vi "PipelineDuty.vi"(8 "error in (no error)":errorcluster, 10 "DataExchange":T1, 11 "GRMActor in":refnum<class "DisplayerUI.lvclass">) -> (0 "error out":errorcluster, 2 "DataExchange Out":T1, 3 "GRMActor out":refnum<class "DisplayerUI.lvclass">)   [LabVIEW 2020, in "DisplayerUI.lvlib" / "DisplayerUI.lvclass"]
uses:
  DisplayerUI.lvclass
  Hardware Abstraction Layer/Component/Device/Device/DataExchange.ctl
  Hardware Abstraction Layer/Component/GenericActor/GenericActor/GenericController.lvclass
  DisplayerUI.lvclass/DisplayerUI.ctl
  Interface/DataListener/DataListener.lvclass
panel:
  out "Source":string
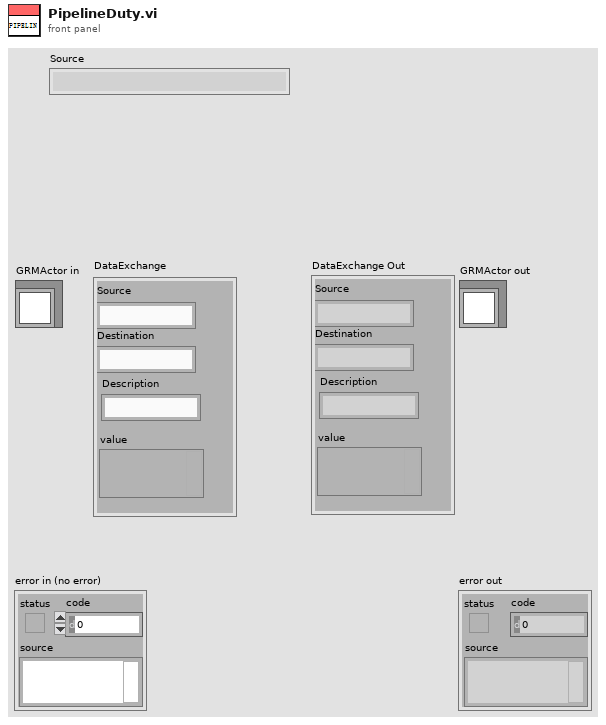
[diagram p1: front panel]
types:
  T1 = typedef "DataListener.lvclass/DataExchange.ctl" = cluster{"Source":string, "Destination":string, "Description":string, "value":variant}
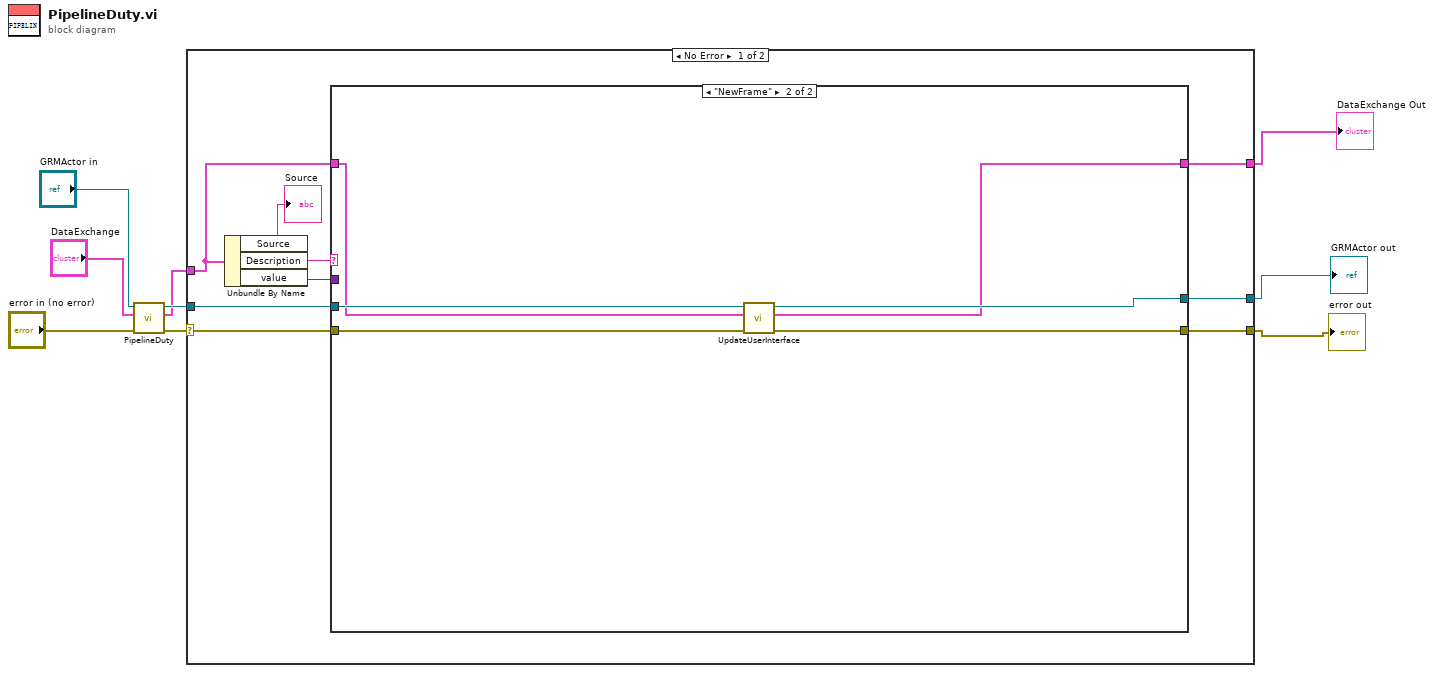
[diagram p0: block diagram]
diagram:
  n1 = call-parent "PipelineDuty.vi"("error in (no error)"="error in (no error)", "DataExchange"="DataExchange", "GRMActor in"="GRMActor in") -> ("error out"=w6:errorcluster, "DataExchange Out"=w4:T1, "GRMActor out"=w5:refnum<class "DisplayerUI.lvclass">)  [unwired: 6 in]
  n2 = case shown="No Error" w6 {
    selector: w6 -> [w16 w30]
    tunnel: [w17 w30] -> w2
    tunnel: w5 -> [w13 w29]
    tunnel: [w18 w29] -> w3
    tunnel: w4 -> [w12 w28]
    tunnel: [w11 w28] -> w1
    frame No Error {
      n3 = Unbundle By Name(w12) -> ("Source"=→"Source":string, "Description"=w15:string, "value"=w14:variant)
      n4 = case shown="\"NewFrame\"" w15 {
        tunnel: w14 -> [_ _]
        tunnel: [w21 w24] -> w18
        tunnel: w13 -> [w21 w25]
        tunnel: [w20 w26] -> w17
        tunnel: w16 -> [w20 w27]
        tunnel: w12 -> [w19 w23]
        tunnel: [w19 w22] -> w11
        frame Default {
        }
        frame "NewFrame" {
          n5 = call-dynamic "UpdateUserInterface.vi"("error in (no error)"=w27, "DataExchange"=w23, "DisplayerUI in"=w25) -> ("error out"=w26:errorcluster, "DataExchange Out"=w22:T1, "DisplayerUI out"=w24:refnum<class "DisplayerUI.lvclass">)  [unwired: 6 in]
        }
      }
    }
    frame Error {
    }
  }
  "error out" <- w2
  "GRMActor out" <- w3
  "DataExchange Out" <- w1
